vi "Code Completion.vi"() -> ()   [LabVIEW 2026]
panel:
  in  "frequency":dbl=60.0
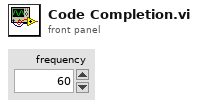
[diagram p1: front panel]
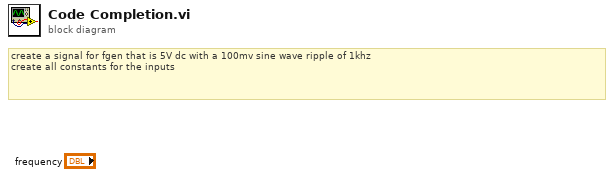
[diagram p0: block diagram]
diagram:
  # "create a signal for fgen that is 5V dc with a 100mv sine wave ripple of 1khz\ncreate all constants for the inputs"
